vi "LCR_Readout.vi"(8 "error in (no error)":errorcluster, 10 "Frequency in Hz":i32, 11 "WK6440B in":refnum<class "WK6440B.lvclass">) -> (0 "error out":errorcluster, 1 "Resistance in Ohm":dbl, 2 "Capacitance in pF":dbl, 3 "WK6440B out":refnum<class "WK6440B.lvclass">)   [LabVIEW 2018, in "WK6440B.lvclass"]
uses:
  WK6440B.lvclass
  C:/Users/itk/Documents/itk-strip-sensor-qc/InstrControl/InstrControl.lvclass
  InstrControl.lvclass
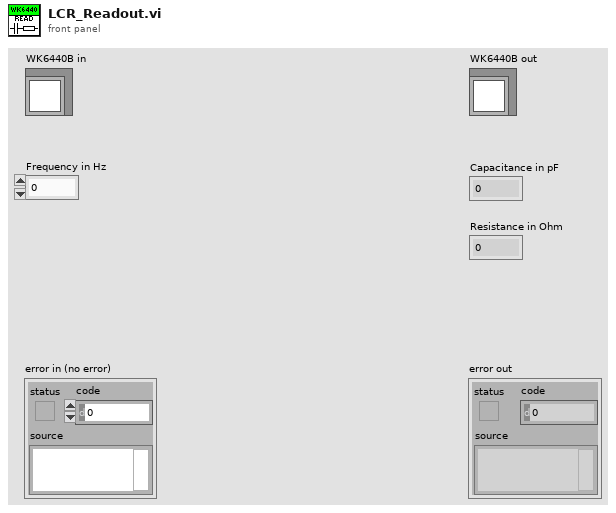
[diagram p1: front panel]
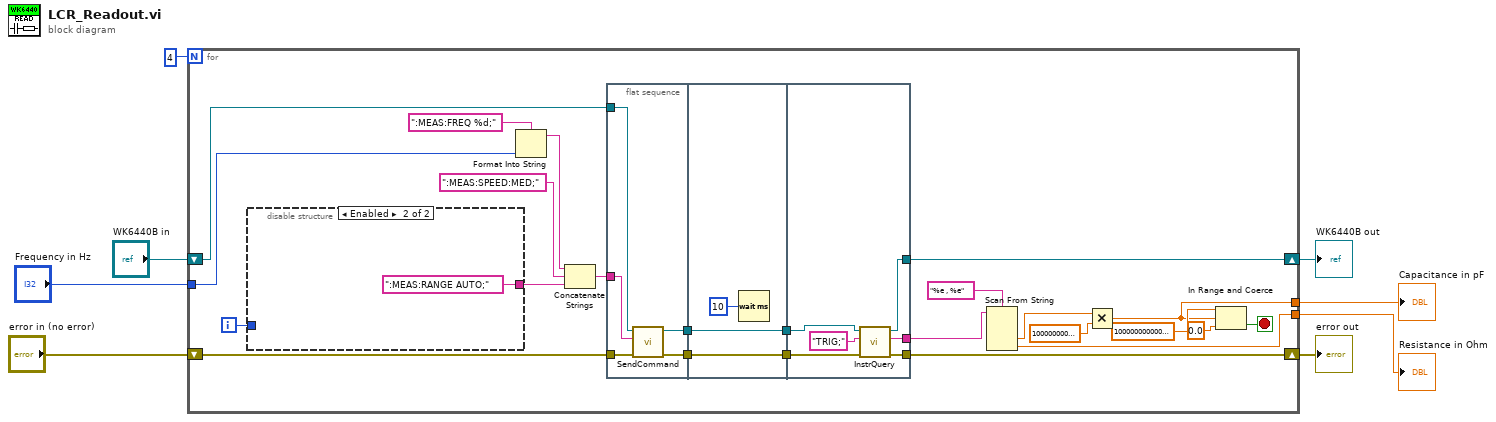
[diagram p0: block diagram]
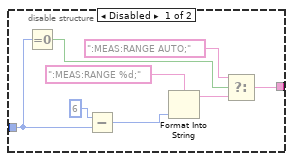
[diagram p2: hidden frame]
diagram:
  n1 = for {
    N: 4 -> [_]
    tunnel: [w9] -> w4
    tunnel: [w29] -> w5
    tunnel: "Frequency in Hz" -> [w26]
    shift-right: [w10] -> w1
    shift-left: "WK6440B in" -> [w17]
    shift-right: [w15] -> w6
    shift-left: "error in (no error)" -> [w25]
    i -> [w28]
    stop <- w27 stop-if-true
    n2 = disable-structure shown="Enabled" {
      disable-tunnel: w28 -> [w40 _]
      disable-tunnel: [w39 ":MEAS:RANGE AUTO;"] -> w21
      frame Disabled {
        n3 = Equal To 0?(x=w40) -> (x = 0?=w35:bool)
        n4 = Subtract(x=6, y=w40) -> (x-y=w33:i32)
        n5 = Format Into String(format string=":MEAS:RANGE %d;", w33) -> (resulting string=w36:string)  [unwired: 2 in, 1 out]
        n6 = Select(t=":MEAS:RANGE AUTO;", s=w35, f=w36) -> (s? t:f=w39:string)
      }
      frame Enabled {
      }
    }
    n7 = Format Into String(format string=":MEAS:FREQ %d;", w26) -> (resulting string=w24:string)  [unwired: 2 in, 1 out]
    n8 = Concatenate Strings(w24, ":MEAS:SPEED:MED;", w21) -> (w32:string)
    n9 = flat-sequence {
      tunnel: w32 -> [w44]
      tunnel: w25 -> [w46]
      tunnel: w17 -> [w42]
      tunnel: [w45] -> w14
      tunnel: [w43] -> w12
      tunnel: w14 -> [w48]
      tunnel: [w48] -> w13
      tunnel: w12 -> [w47]
      tunnel: [w47] -> w11
      tunnel: [w54] -> w15
      tunnel: [w53] -> w16
      tunnel: w13 -> [w55]
      tunnel: w11 -> [w51]
      tunnel: [w50] -> w10
      frame #0 {
        n10 = call "SendCommand.vi"("error in (no error)"=w46, "Command string"=w44, "InstControl in"=w42) -> ("error out"=w45:errorcluster, "InstControl out"=w43:refnum<class "WK6440B.lvclass">)  [unwired: 7 in]
      }
      frame #1 {
        n11 = Wait (ms)(milliseconds to wait=10) -> ()  [unwired: 1 out]
      }
      frame #2 {
        n12 = call-dynamic "InstrQuery.vi"("error in (no error)"=w55, "Command string"="TRIG;", "InstControl in"=w51) -> ("error out"=w54:errorcluster, "Instrument response"=w53:string, "InstControl out"=w50:refnum<class "WK6440B.lvclass">)  [unwired: 6 in]
      }
    }
    n13 = Scan From String(format string="%e , %e", input string=w16) -> (output 1=w18:dbl, output 2=w9:dbl)  [unwired: 4 in, 3 out]
    n14 = Multiply(x=w18, y=1000000000000.0) -> (x*y=w29:dbl)
    n15 = In Range and Coerce(upper limit=100000000000000.0 ("y"), x=w29, lower limit=0.0) -> (In Range?=w27:bool)  [unwired: 1 out]
  }
  "error out" <- w6
  "WK6440B out" <- w1
  "Capacitance in pF" <- w5
  "Resistance in Ohm" <- w4
